vi "hse-configuration_ParseConfigSource.vi"(8 "error in (no error)":errorcluster, 10 "Config Source":variant, 11 "hse-configuration in":refnum<class "hse-configuration.lvclass">) -> (0 "error out":errorcluster, 3 "hse-configuration out":refnum<class "hse-configuration.lvclass">)   [LabVIEW 2014, in "hse-configuration.lvclass"]
doc: "Parses the configuration source and stores the contents in memory for future use.\n\n____\nHAMPEL SOFTWARE ENGINEERING v0.12.0 (2018-09-13 18:21)"
uses:
  hse-configuration.lvclass
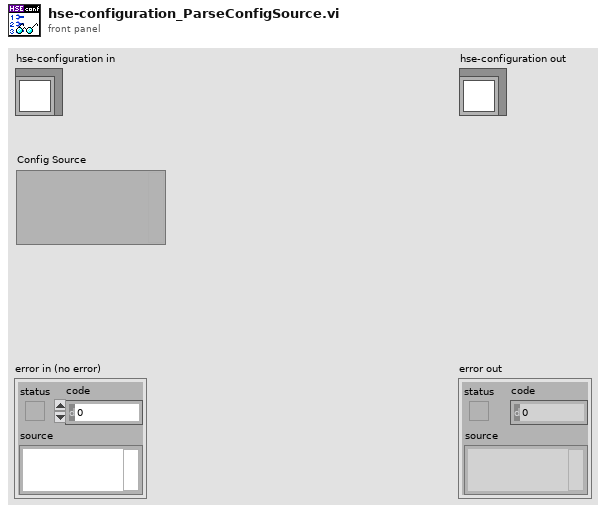
[diagram p1: front panel]
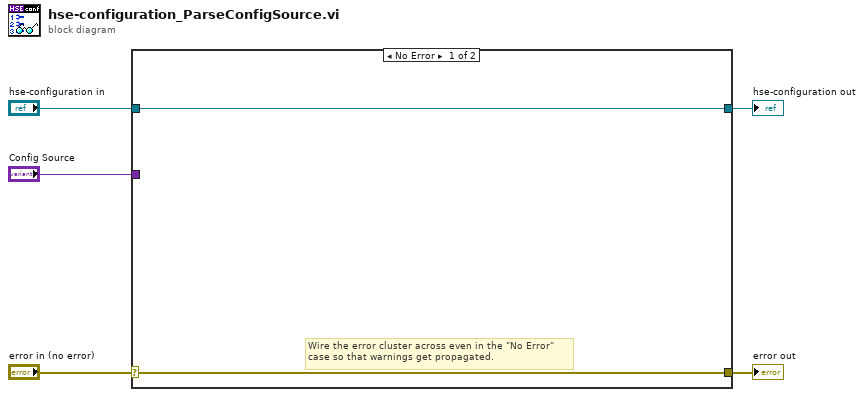
[diagram p0: block diagram]
diagram:
  n1 = case shown="No Error" "error in (no error)" {
    selector: "error in (no error)" -> [w6 w9]
    tunnel: [w6 w9] -> w4
    tunnel: [w7 w8] -> w2
    tunnel: "hse-configuration in" -> [w7 w8]
    tunnel: "Config Source" -> [_ _]
    frame No Error {
      # "Wire the error cluster across even in the \"No Error\"\ncase so that warnings get propagated."
    }
    frame Error {
    }
  }
  "error out" <- w4
  "hse-configuration out" <- w2
